vi "CreateAllQueue.vi"() -> (0 "error out":errorcluster, 3 "Queue cluster":T1)   [LabVIEW 2017]
uses:
  QueueCluster.ctl
  EventQueueCluster.ctl
  EventMessage.ctl
  MeasureQueue.ctl
  MeasureMessage.ctl
  HardwareQueueCluster.ctl
  hardwareMessage.ctl
  GUIQueueCluster.ctl
  GUIMessage.ctl
  SaveQueueCluster.ctl
  SaveMessage.ctl
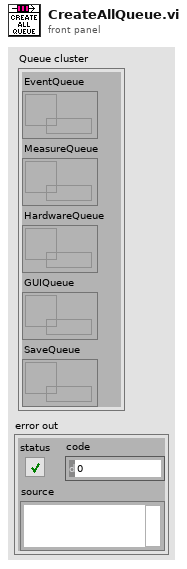
[diagram p1: front panel]
types:
  T1 = typedef "QueueCluster.ctl" = cluster{"EventQueue":refnum<queue>, "MeasureQueue":refnum<queue>, "HardwareQueue":refnum<queue>, "GUIQueue":refnum<queue>, "SaveQueue":refnum<queue>}
  T2 = cluster{"EventQueue":refnum<queue>, "MeasureQueue":refnum<queue>, "HardwareQueue":refnum<queue>, "GUIQueue":refnum<queue>, "Save queue":refnum<queue>}
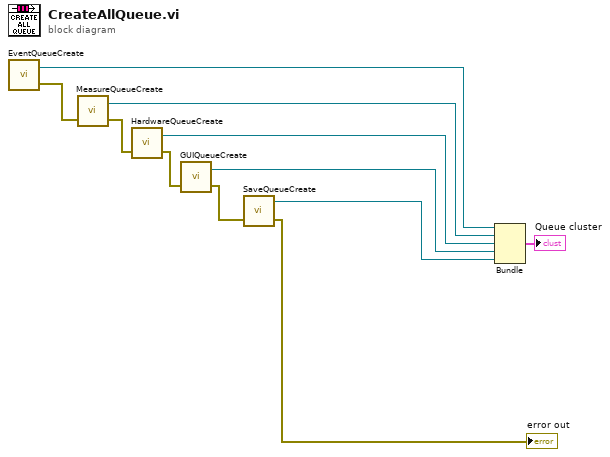
[diagram p0: block diagram]
diagram:
  n1 = call "EventQueueCreate.vi"() -> ("EventError"=w10:errorcluster, "EventQueue"=w7:refnum<queue>)  [unwired: 2 in]
  n2 = call "MeasureQueueCreate.vi"("error in (no error)"=w10) -> ("MeasureError"=w11:errorcluster, "MeasureQueue"=w8:refnum<queue>)  [unwired: 1 in]
  n3 = call "HardwareQueueCreate.vi"("error in (no error)"=w11) -> ("HardwareError"=w6:errorcluster, "HardwareQueue"=w9:refnum<queue>)  [unwired: 1 in]
  n4 = call "GUIQueueCreate.vi"("error in (no error)"=w6) -> ("GUIError"=w5:errorcluster, "GUIQueue"=w4:refnum<queue>)  [unwired: 1 in]
  n5 = call "SaveQueueCreate.vi"("error in (no error)"=w5) -> ("error out"=→"error out":errorcluster, "Save queue"=w2:refnum<queue>)  [unwired: 1 in]
  n6 = Bundle("EventQueue"=w7, "MeasureQueue"=w8, "HardwareQueue"=w9, "GUIQueue"=w4, "Save queue"=w2) -> (→"Queue cluster":T2)  [unwired: 1 in]
